vi "Image UDP Broadcast Global Variable.vi"() -> ()   [LabVIEW 2012, in "Image UDP Broadcast Custom Device.lvlib"]
uses:
  Image UDP Broadcast Custom Device.lvlib
panel:
  in  "IP Address":string="IP Address"
  in  "Max BpP":i32=8192
  in  "Camera Interface":string="Camera Interface"
  in  "Image Type":string="Image Type"
  in  "Quality":string="Quality"
  in  "UDP Port":string="UDP Port"
  in  "Bytes per Packet":string="Bytes per Packet"
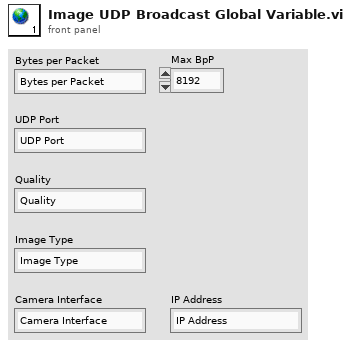
[diagram p1: front panel]
diagram:
